vi "SQLAllocHandle.vi"(4 "error in (no error)":errorcluster, 6 "HandleType":T1(ring)=enum."SQL_HANDLE_ENV", 7 "InputHandle":i32) -> (0 "error out":errorcluster, 3 "OutputHandle":i32)   [LabVIEW 2011]
doc: "Fournit un lien de type environnement, ODBC, requête..."
uses:
  Odbc32.dll
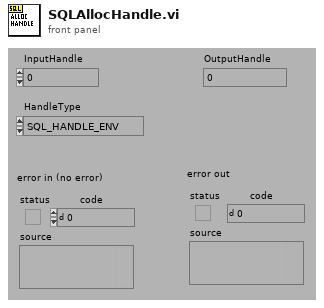
[diagram p1: front panel]
types:
  T1 = enum16{"NOPE", "SQL_HANDLE_ENV", "SQL_HANDLE_DBC", "SQL_HANDLE_STMT", "SQL_HANDLE_DESC"}
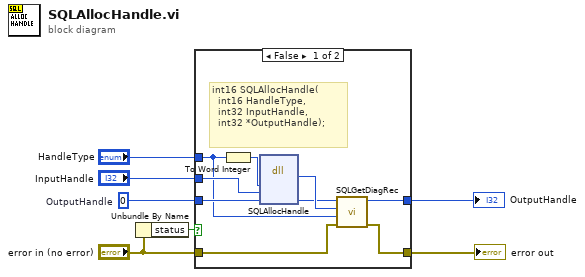
[diagram p0: block diagram]
diagram:
  w6 = 0  # OutputHandle
  n1 = Unbundle By Name("error in (no error)") -> ("status"=w4:bool)
  n2 = case shown="False" w4 {
    tunnel: "InputHandle" -> [w16 _]
    tunnel: w6 -> [w15 w17]
    tunnel: "HandleType" -> [w8 _]
    tunnel: [w12 w18] -> w2
    tunnel: "error in (no error)" -> [w13 w18]
    tunnel: [w10 w17] -> w1
    frame False {
      # "int16 SQLAllocHandle(\n  int16 HandleType, \n  int32 InputHandle, \n  int32 *OutputHandle);"
      n3 = To Word Integer(number=w8) -> (16bit integer=w9:i16)
      n4 = dll-call lib="Odbc32.dll" fn="SQLAllocHandle"("HandleType"=w9, "InputHandle"=w16, "OutputHandle"=w15) -> (w14:i16, "OutputHandle"=w11:i32)  [unwired: 5 in, 2 out]
      n5 = call "SQLGetDiagRec.vi"("error in (no error)"=w13, "HandleType"=w8, "Status (SQL_SUCCESS=0)"=w14, "Input Handle"=w11) -> ("error out"=w12:errorcluster, "Output Handle"=w10:i32)  [unwired: 2 out]
    }
    frame True {
    }
  }
  "error out" <- w2
  "OutputHandle" <- w1
